vi "1 channel 1 sample temp.vi"() -> ()   [LabVIEW 2020]
uses:
  <vilib>/DAQmx/read.llb/DAQmx Read (Analog DBL 1Chan 1Samp).vi
  <vilib>/DAQmx/create/channels.llb/DAQmx Create Channel (AI-Temperature-Thermocouple).vi
  <vilib>/DAQmx/configure/timing.llb/DAQmx Timing (Sample Clock).vi
  <vilib>/DAQmx/miscellaneous.llb/DAQmx Fill In Error Info.vi
panel:
  out "data":dbl format="%0.2f"
  in  "file path (use dialog)":path
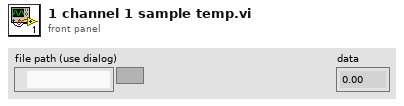
[diagram p1: front panel]
types:
  T1 = enum16{"open", "replace", "create", "open or create", "replace or create", "replace or create with confirmation"}
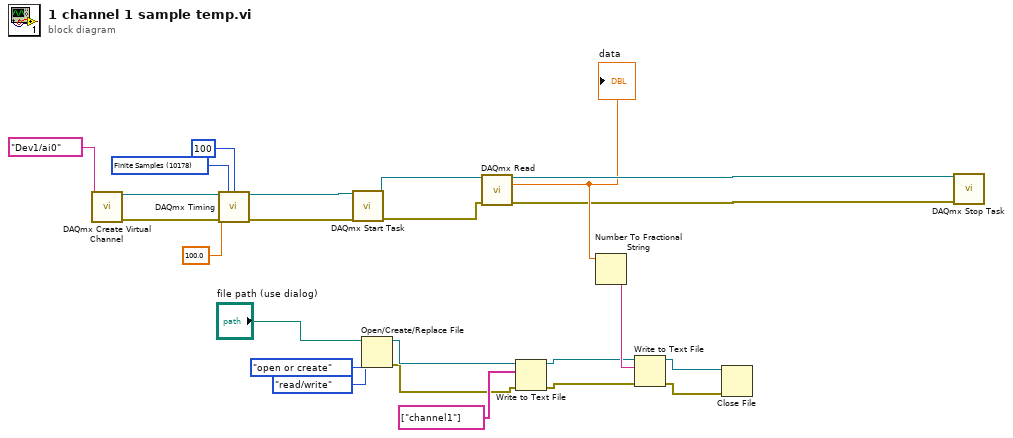
[diagram p0: block diagram]
diagram:
  w5 = 10178 items=["Finite Samples"=10178, "Continuous Samples"=10123, "Hardware Timed Single Point"=12522] ("sample mode")
  n1 = call-poly <vilib>:"DAQmx Create Virtual Channel.vi"("physical channels"=tag "Dev1/ai0") -> ("task out"=w24:refnum<k21>, "error out"=w20:errorcluster)  [unwired: 13 in]
  n2 = call-poly <vilib>:"DAQmx Timing.vi"("task/channels in"=w24, "sample mode"=w5, "samples per channel"=100, "rate"=100.0, "error in"=w20) -> ("task out"=w23:refnum<k21>, "error out"=w19:errorcluster)  [unwired: 9 in]
  n3 = call <vilib>:"DAQmx Start Task.vi"("task/channels in"=w23, "error in"=w19) -> ("task out"=w22:refnum<k21>, "error out"=w18:errorcluster)  [unwired: 12 in]
  n4 = Open/Create/Replace File(file path (use dialog)="file path (use dialog)", operation (0:open)=T1."open or create", access (0:read/write)=enum16{"read/write", "read-only", "write-only"}."read/write") -> (refnum out=w12:refnum<file>, error out=w11:errorcluster)  [unwired: 3 in, 1 out]
  n5 = call-poly <vilib>:"DAQmx Read.vi"("task/channels in"=w22, "error in"=w18) -> ("task out"=w21:refnum<k21>, "data"=w17:dbl, "error out"=w2:errorcluster)  [unwired: 11 in]
  "data" <- w17
  n6 = Write to Text File(file (use dialog)=w12, text=string[] ["channel1"], error in=w11) -> (refnum out=w14:refnum<file>, error out=w10:errorcluster)  [unwired: 1 in, 1 out]
  n7 = Number To Fractional String(number=w17) -> (F-format string=w16:string)  [unwired: 3 in]
  n8 = Write to Text File(file (use dialog)=w14, text=w16, error in=w10) -> (refnum out=w13:refnum<file>, error out=w9:errorcluster)  [unwired: 1 in, 1 out]
  n9 = Close File(refnum=w13, error in=w9) -> ()  [unwired: 2 out]
  n10 = call <vilib>:"DAQmx Stop Task.vi"("task/channels in"=w21, "error in"=w2) -> ()  [unwired: 12 in, 2 out]
